vi "digitDisplay.vi"(1 "Numeric":i32) -> (0 "new picture":picture)   [LabVIEW 2024]
panel:
  out "Ring":u16(ring)
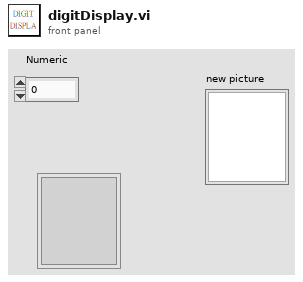
[diagram p1: front panel]
types:
  T1 = typedef "imagedata.ctl" = cluster{"image type":i32, "image depth":i32, "image":u8[], "mask":u8[], "colors":u32[], "Rectangle":cluster{"left":i16, "top":i16, "right":i16, "bottom":i16}}
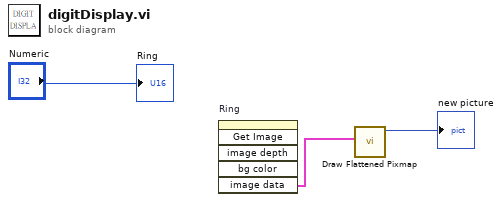
[diagram p0: block diagram]
diagram:
  n1 = invoke on="Ring" class="Ring (strict)" method="Get Image"() -> ("image data"=w3:T1)  [unwired: 6 in, 5 out]
  n2 = call <vilib>:"Draw Flattened Pixmap.vi"("image data"=w3) -> ("new picture"=→"new picture":picture)  [unwired: 8 in]
  "Ring" <- "Numeric"
